vi "Ex10.vi"() -> ()   [LabVIEW 2016]
panel:
  out "Loop 2":i32
  out "Loop 1":i32
  in  "정지":bool
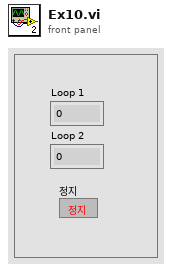
[diagram p1: front panel]
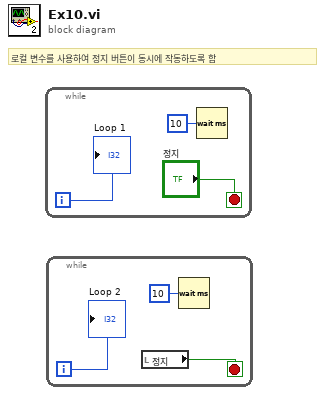
[diagram p0: block diagram]
diagram:
  # "로컬 변수를 사용하여 정지 버튼이 동시에 작동하도록 함"
  n1 = while {
    i -> [w2]
    stop <- "정지" stop-if-true
    n2 = Wait (ms)(milliseconds to wait=u32 10 ("대기 시간 (ms)")) -> ()  [unwired: 1 out]
    "Loop 1" <- w2
  }
  n3 = while {
    i -> [w5]
    stop <- w6 stop-if-true
    n4 = local read "정지"() -> (w6:bool)
    n5 = Wait (ms)(milliseconds to wait=u32 10 ("대기 시간 (ms)")) -> ()  [unwired: 1 out]
    "Loop 2" <- w5
  }
